vi "Get RX Message.vi"(8 "error in (no error)":errorcluster, 11 "RxTx in":refnum<class "RxTx.lvclass">) -> (0 "error out":errorcluster, 3 "RxTx out":refnum<class "RxTx.lvclass">)   [LabVIEW 2018, in "RxTx.lvclass"]
uses:
  RxTx.lvclass
  RxTx.lvclass/RxTx.ctl
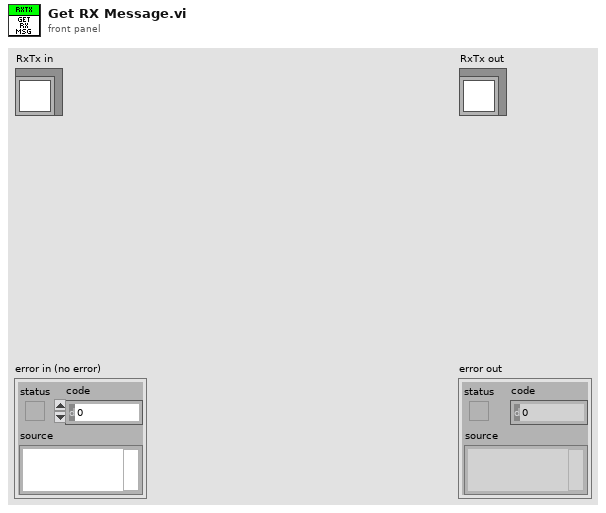
[diagram p1: front panel]
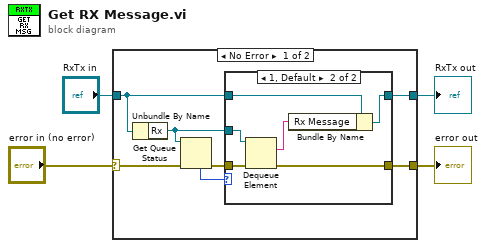
[diagram p0: block diagram]
diagram:
  n1 = case shown="No Error" "error in (no error)" {
    selector: "error in (no error)" -> [w7 w21]
    tunnel: [w5 w21] -> w1
    tunnel: [w10 w20] -> w2
    tunnel: "RxTx in" -> [w11 w20]
    frame No Error {
      n2 = Unbundle By Name(w11) -> ("Rx"=w8:refnum<queue>)
      n3 = Get Queue Status(queue=w8, error in (no error)=w7) -> (error out=w6:errorcluster, # elements in queue=w9:i32)  [unwired: 1 in, 6 out]
      n4 = case shown="1, Default" w9 {
        tunnel: w8 -> [_ w19]
        tunnel: w11 -> [w12 w18]
        tunnel: [w12 w17] -> w10
        tunnel: w6 -> [w13 w15]
        tunnel: [w13 w14] -> w5
        frame 0 {
        }
        frame 1, Default {
          n5 = Dequeue Element(queue=w19, error in (no error)=w15) -> (element=w16:string, error out=w14:errorcluster)  [unwired: 1 in, 2 out]
          n6 = Bundle By Name(cluster=w18, "Rx Message"=w16) -> (w17:refnum<class "RxTx.lvclass">)
        }
      }
    }
    frame Error {
    }
  }
  "error out" <- w1
  "RxTx out" <- w2
